vi "Instantiate.vi"(1 "vi ref":refnum<vi>) -> (0 "vi ref":refnum<vi>)   [LabVIEW 2019, in "Cmd-Data Event Messenger.lvlib"]
doc: "Creates and initializes the data structure that supports the channel at run time."
uses:
  Cmd-Data Event Messenger.lvlib
  ))Channel.vi
  ChannelOp.ctl
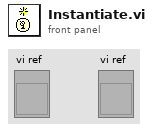
[diagram p1: front panel]
types:
  T1 = typedef "Cmd-Data Event Messenger.lvlib/ChannelOp.ctl" = enum16{"init", "write", "register", "replicate", "probe"}
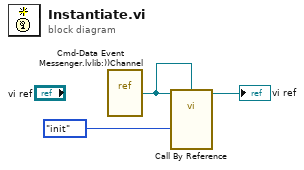
[diagram p0: block diagram]
diagram:
  n1 = vi-ref "Cmd-Data Event Messenger.lvlib:))Channel.vi"() -> (w1:refnum<vi>)
  n2 = call-by-ref "?"(reference=w1, "This VI"=w1, "channelOp"=ChannelOp."init") -> (reference out=→"vi ref":refnum<vi>)  [unwired: 10 in, 6 out]
